vi "keyboard.vi"   [LabVIEW 2020]
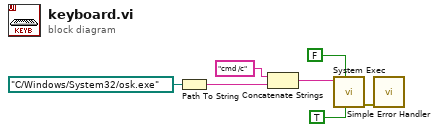
[diagram p0: block diagram]
diagram:
  n1 = Path To String(path=path "C:/Windows/System32/osk.exe") -> (string=w6:string)
  n2 = Concatenate Strings("cmd /c" ("string"), w6) -> (w4:string)
  n3 = call <vilib>:"System Exec.vi"("run minimized? (F)"=TRUE, "wait until completion? (T)"=FALSE, "command line"=w4) -> ("error out"=w2:errorcluster)  [unwired: 5 in, 3 out]
  n4 = call <vilib>:"Simple Error Handler.vi"("error in (no error)"=w2) -> ()  [unwired: 4 in, 5 out]
